vi "Self Test.vi"(8 "error in":errorcluster, 11 "6509 in":refnum<class "6509.lvclass">) -> (0 "error out":errorcluster, 3 "6509 out":refnum<class "6509.lvclass">)   [LabVIEW 2019, in "6509.lvlib" / "6509.lvclass"]
uses:
  Library/6509.lvclass
  C:/Users/Public/Documents/Development/builds/Instruments/DIG_IO.lvlibp/Library/DIG_IO.lvclass
  Library/6509.lvclass/6509.ctl
  builds/Instruments/DIG_IO.lvlibp/Accessors/Read IO_Mode.vi
  builds/Instruments/DIG_IO.lvlibp/Library/DIG_IO.lvclass
  <resource>/objmgr/daqmx.rc
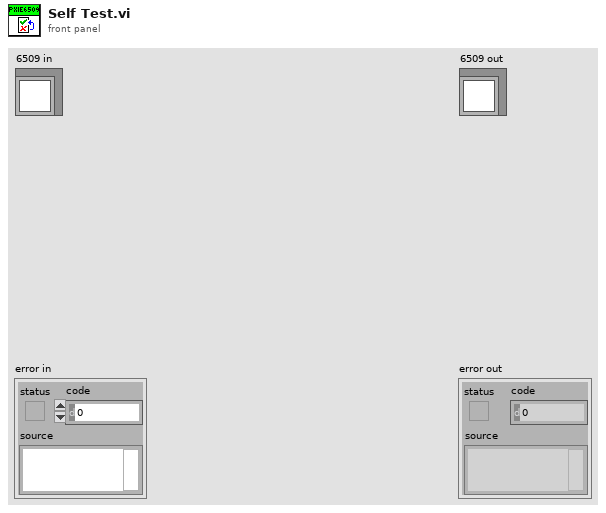
[diagram p1: front panel]
types:
  T1 = typedef "DIG_IO.lvlibp/DIG_IO.lvclass/IO Mode.ctl" = enum16{"IO", "IN", "OUT"}
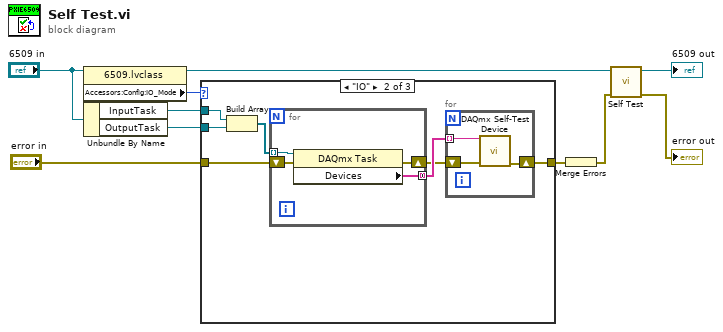
[diagram p0: block diagram]
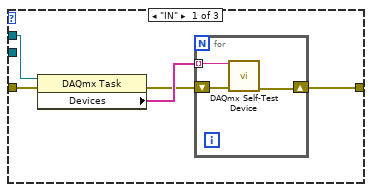
[diagram p2: hidden frame]
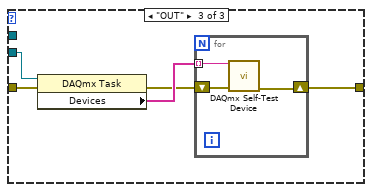
[diagram p3: hidden frame]
diagram:
  n1 = property class="6509.lvclass"(reference="6509 in") -> (reference out=w2:refnum<class "6509.lvclass">, "Accessors:Config:IO_Mode"=w1:T1)  [unwired: 1 in, 1 out]
  n2 = Unbundle By Name("6509 in") -> ("InputTask"=w5:refnum<k21>, "OutputTask"=w4:refnum<k21>)
  n3 = case shown="\"IO\"" w1 {
    tunnel: [w15 w25 w37] -> w9
    tunnel: "error in" -> [w14 w24 w36]
    tunnel: w5 -> [w11 w21 _]
    tunnel: w4 -> [_ w20 w33]
    frame "IN" {
      n4 = property class="DAQmx Task"(reference=w11, error in=w14) -> (error out=w12:errorcluster, "Devices"=w13:tag[])  [unwired: 1 out]
      n5 = for {
        tunnel: w13 -> [w18] mode=indexing
        shift-right: [w16] -> w15
        shift-left: w12 -> [w17]
        n6 = call <vilib>:"DAQmx Self-Test Device.vi"("device in"=w18, "error in"=w17) -> ("error out"=w16:errorcluster)  [unwired: 13 in]
      }
    }
    frame "IO" {
      n7 = Build Array(w21, w20) -> (w19:refnum<k21>[])
      n8 = for {
        tunnel: [w28] -> w23 mode=concatenating
        shift-right: [w27] -> w22
        shift-left: w24 -> [w29]
        tunnel: w19 -> [w26] mode=indexing
        n9 = property class="DAQmx Task"(reference=w26, error in=w29) -> (error out=w27:errorcluster, "Devices"=w28:tag[])  [unwired: 1 out]
      }
      n10 = for {
        tunnel: w23 -> [w32] mode=indexing
        shift-right: [w30] -> w25
        shift-left: w22 -> [w31]
        n11 = call <vilib>:"DAQmx Self-Test Device.vi"("device in"=w32, "error in"=w31) -> ("error out"=w30:errorcluster)  [unwired: 13 in]
      }
    }
    frame "OUT" {
      n12 = property class="DAQmx Task"(reference=w33, error in=w36) -> (error out=w34:errorcluster, "Devices"=w35:tag[])  [unwired: 1 out]
      n13 = for {
        tunnel: w35 -> [w40] mode=indexing
        shift-right: [w38] -> w37
        shift-left: w34 -> [w39]
        n14 = call <vilib>:"DAQmx Self-Test Device.vi"("device in"=w40, "error in"=w39) -> ("error out"=w38:errorcluster)  [unwired: 13 in]
      }
    }
  }
  n15 = Merge Errors(w9) -> (w6:errorcluster)
  n16 = call-parent "Self Test.vi"("error in"=w6, "Instruments in"=w2) -> ("error out"=→"error out":errorcluster, "Instruments out"=→"6509 out":refnum<class "6509.lvclass">)  [unwired: 8 in]
